vi "Write SkipTabbing.vi"(5 "SkipTabbing":bool, 9 "Control in":refnum<class "Control.lvclass">) -> (3 "Control out":refnum<class "Control.lvclass">)   [LabVIEW 2014, in "Control.lvclass"]
uses:
  Control.lvclass
  Control.lvclass/Control.ctl
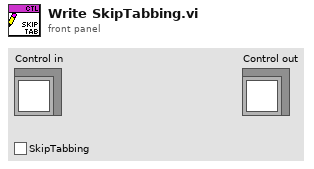
[diagram p1: front panel]
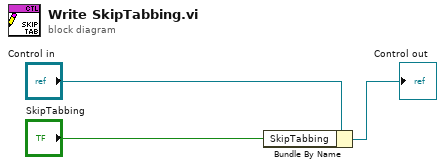
[diagram p0: block diagram]
diagram:
  n1 = Bundle By Name(cluster="Control in", "SkipTabbing"="SkipTabbing") -> (→"Control out":refnum<class "Control.lvclass">)
